vi "Day 3.vi"() -> ()   [LabVIEW 2021]
panel:
  out "input":string
  out "input file":path
  out "ouptut part 2":u64
  in  "Run [T]/ Example[F]":bool
  out "ouptut part 1":u64
  # "Advent of Code 2023 - Day 3 - Gear Ratios"
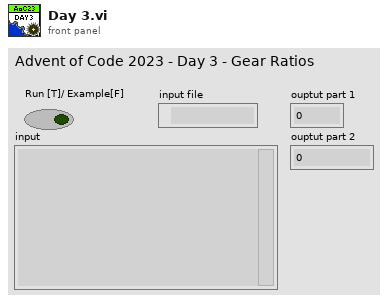
[diagram p1: front panel]
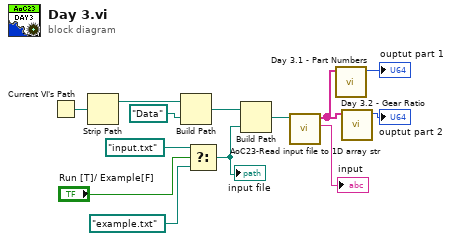
[diagram p0: block diagram]
diagram:
  n1 = Current VI's Path() -> (path=w13:path)
  n2 = Strip Path(path=w13) -> (stripped path=w12:path)  [unwired: 1 out]
  n3 = Build Path(base path=w12, name or relative path=path "Data") -> (appended path=w10:path)
  n4 = Select(t=path "input.txt" ("name or relative path"), s="Run [T]/ Example[F]", f=path "example.txt" ("name or relative path")) -> (s? t:f=w6:path)
  "input file" <- w6
  n5 = Build Path(base path=w10, name or relative path=w6) -> (appended path=w5:path)
  n6 = call "AoC23-Read input file to 1D array str.vi"("input file"=w5) -> ("input text"=→"input":string, "input"=w1:string[])  [unwired: 9 in]
  n7 = call "Day 3.1 - Part Numbers.vi"("input"=w1) -> ("ouptut part 1"=→"ouptut part 1":u64)  [unwired: 10 in]
  n8 = call "Day 3.2 - Gear Ratio.vi"("input"=w1) -> ("ouptut part 2"=→"ouptut part 2":u64)  [unwired: 10 in]
